vi "Apply Poly Fit.vi"(10 "Data In":dbl[](array[numeric]), 11 "Polynomial Coefficients":dbl[](array[numeric])) -> (3 "Data Out":dbl[](array[numeric]))   [LabVIEW 2017]
uses:
  <vilib>/Analysis/polynomials.llb/Scalar Polynomial Evaluation (DBL).vi
  <vilib>/Analysis/NI_AALPro.lvlib
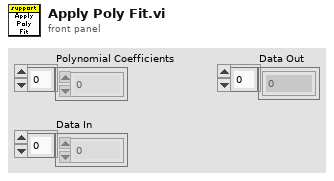
[diagram p1: front panel]
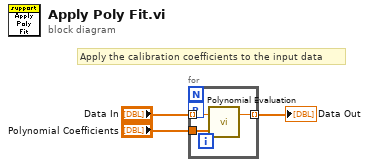
[diagram p0: block diagram]
diagram:
  # "Apply the calibration coefficients to the input data"
  n1 = for {
    tunnel: "Polynomial Coefficients" -> [w6]
    tunnel: "Data In" -> [w5] mode=indexing
    tunnel: [w4] -> w3 mode=indexing
    workers-P: _ -> [_]
    n2 = call-poly <vilib>:"Polynomial Evaluation.vi"("P(x)"=w6, "a"=w5) -> ("P(a)"=w4:dbl)  [unwired: 1 out]
  }
  "Data Out" <- w3
